vi "Set Columns.vi"(8 "Error In":errorcluster, 10 "<JSON> Columns Definition in":string, 11 "object in":refnum<class "Component.Tabulator.lvclass">) -> (0 "Error Out":errorcluster, 3 "object out":refnum<class "Component.Tabulator.lvclass">)   [LabVIEW 2020, in "Component.Tabulator.lvclass"]
uses:
  Component.Tabulator.lvclass
  <vilib>/JDP Science/JSONtext/LVClass Serializer/JSONtext LVClass Serializer.lvclass
  <vilib>/sklein/WebView2/Webview2 Lib/WebView2 Control Object/WebView2 Control.lvclass
  e4739fd8-f072-441e-97c6-a5a89ce9ff40.vi
  Message Types--enum.ctl
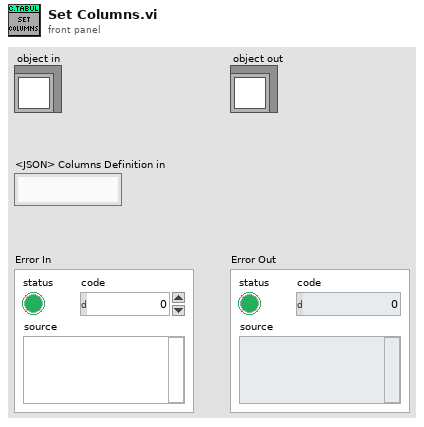
[diagram p1: front panel]
types:
  T1 = typedef "Component.Tabulator.lvclass/Message Types--enum.ctl" = enum16{"loadData", "setColumns", "getData", "addRow", "deleteRow", "updateRow", "clearData", "downloadCSV", "downloadJSON", "print", "selectRow", "deselectRow", "getSelectedRows", "redraw"}
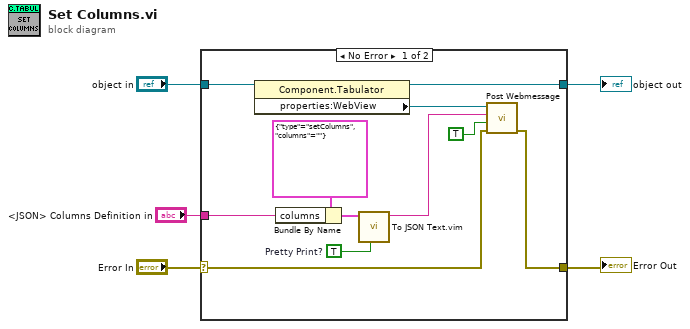
[diagram p0: block diagram]
diagram:
  n1 = case shown="No Error" "Error In" {
    selector: "Error In" -> [w8 w18]
    tunnel: [w6 w18] -> w4
    tunnel: [w10 w17] -> w2
    tunnel: "object in" -> [w16 w17]
    tunnel: "<JSON> Columns Definition in" -> [w13 _]
    frame No Error {
      w12 = TRUE  # Pretty Print?
      n2 = property class="Component.Tabulator"(reference=w16) -> (reference out=w10:refnum<class "Component.Tabulator.lvclass">, "properties:WebView"=w11:refnum<class "WebView2 Control.lvclass">)  [unwired: 1 in, 1 out]
      n3 = Bundle By Name(cluster=cluster{"type":T1, "columns":string} {"type"=enum."setColumns", "columns"=""}, "columns"=w13) -> (w14:cluster{"type":T1, "columns":string})
      n4 = call "To JSON Text.vim"("Pretty Print?"=w12, "Anything"=w14) -> ("<JSON>"=w9:string)  [unwired: 8 in, 1 out]
      n5 = call <vilib>:"Post Webmessage.vi"("error in (no error)"=w8, "Send as JSON"=TRUE ("Fetch Result? (T)"), "Message"=w9, "WebView2 Control in"=w11) -> ("error out"=w6:errorcluster)  [unwired: 6 in, 1 out]
    }
    frame Error {
    }
  }
  "Error Out" <- w4
  "object out" <- w2
